vi "Receive Message.vi"(6 "priority":i32, 10 "State Machine in":refnum<class "State Machine.lvclass">, 11 "Message in":refnum<class "Message.lvclass">) -> (0 "error out":errorcluster, 2 "Actor out":refnum<class "Actor.lvclass">)   [LabVIEW 2024, in "State Pattern Actor.lvlib" / "State Machine.lvlib" / "State Machine.lvclass"]
doc: "This VI should be overriden ONLY if you are creating a proxy actor for remote transmission. If you are, override this VI to transmit the received message to a new destination, maintaining the given priority."
uses:
  State Machine.lvclass
  State Machine.lvclass/State Machine.ctl
  <vilib>/ActorFramework/Actor/Actor.lvclass
  <vilib>/ActorFramework/Self-Addressed Msg/Self-Addressed Msg.lvclass
  C:/Program Files (x86)/National Instruments/LabVIEW 2024/vi.lib/ActorFramework/Actor/Actor.lvclass
  C:/Users/uspoaotto/OneDrive - Oregon Tool/Desktop/working copies/stateMachineActor/src/State Pattern Actor/State Machine Actor/State Machine.lvclass
  <vilib>/ActorFramework/Message/Message.lvclass
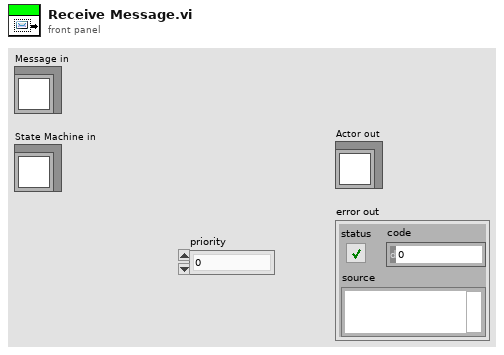
[diagram p1: front panel]
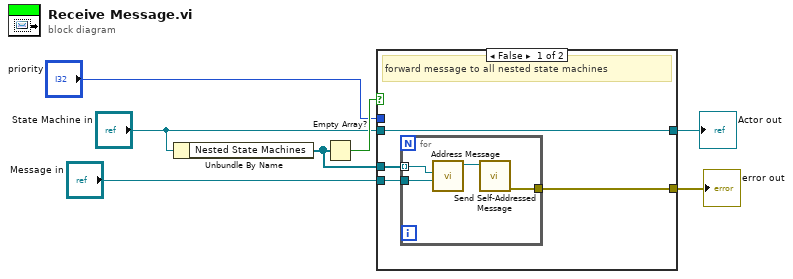
[diagram p0: block diagram]
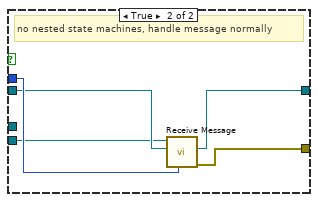
[diagram p2: hidden frame]
diagram:
  n1 = Unbundle By Name("State Machine in") -> ("Nested State Machines"=w1:refnum<class "Message Enqueuer.lvclass">[])
  n2 = Empty Array?(array=w1) -> (empty?=w7:bool)
  n3 = case shown="False" w7 {
    tunnel: "priority" -> [_ w20]
    tunnel: "State Machine in" -> [w11 w19]
    tunnel: "Message in" -> [w9 w18]
    tunnel: [w8 w17] -> w3
    tunnel: [w11 w16] -> w2
    tunnel: w1 -> [w10 _]
    frame False {
      # "forward message to all nested state machines"
      n4 = for {
        tunnel: w10 -> [w15] mode=indexing
        tunnel: w9 -> [w14]
        tunnel: [w12] -> w8
        n5 = call <vilib>:"Address Message.vi"("Message"=w14, "Destination"=w15) -> ("Self-Addressed Message"=w13:refnum<class "Self-Addressed Msg.lvclass">)  [unwired: 9 in]
        n6 = call-dynamic "Send Self-Addressed Message.vi"("Self-Addressed Message in"=w13) -> ("error out"=w12:errorcluster)  [unwired: 9 in, 1 out]
      }
    }
    frame True {
      # "no nested state machines, handle message normally"
      n7 = call-parent "Receive Message.vi"("priority"=w20, "Actor in"=w19, "Message in"=w18) -> ("error out"=w17:errorcluster, "Actor out"=w16:refnum<class "Actor.lvclass">)  [unwired: 7 in]
    }
  }
  "error out" <- w3
  "Actor out" <- w2
